vi "ReceiveString.vi"(8 "error in (no error)":errorcluster, 11 "queue cluster":T1) -> (0 "error out":errorcluster, 1 "new value":bool, 2 "received string":string, 3 "queue cluster out":T1)   [LabVIEW 2014]
uses:
  typedefs/clientStatus.ctl
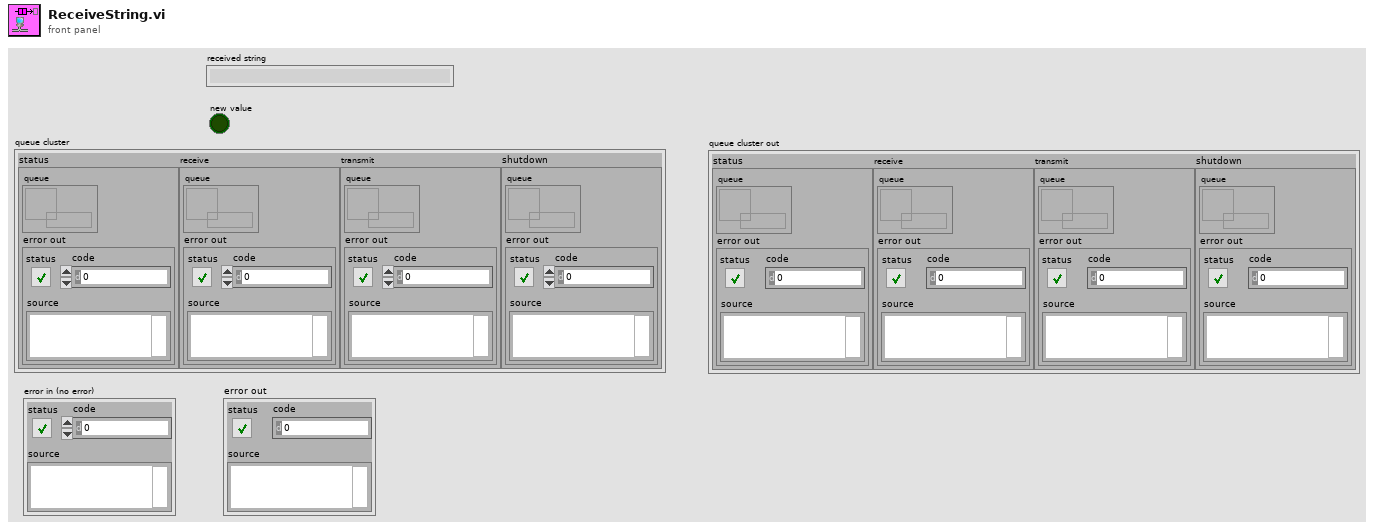
[diagram p1: front panel]
types:
  T1 = cluster{"status":cluster{"queue":refnum<queue>, "error out":errorcluster}, "receive":cluster{"queue":refnum<queue>, "error out":errorcluster}, "transmit":cluster{"queue":refnum<queue>, "error out":errorcluster}, "shutdown":cluster{"queue":refnum<queue>, "error out":errorcluster}}
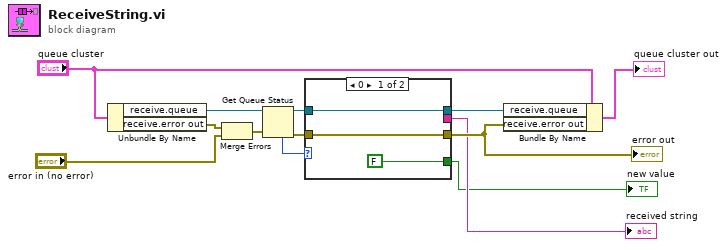
[diagram p0: block diagram]
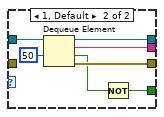
[diagram p2: hidden frame]
diagram:
  n1 = Unbundle By Name("queue cluster") -> ("receive.queue"=w9:refnum<queue>, "receive.error out"=w6:errorcluster)
  n2 = Merge Errors(w6, "error in (no error)") -> (w7:errorcluster)
  n3 = Get Queue Status(queue=w9, error in (no error)=w7) -> (queue out=w8:refnum<queue>, error out=w4:errorcluster, # elements in queue=w3:i32)  [unwired: 1 in, 5 out]
  n4 = case shown="0" w3 {
    tunnel: [w15 w23] -> w11
    tunnel: [w16 w22] -> w10
    tunnel: [_ w21] -> w2
    tunnel: w8 -> [w16 w20]
    tunnel: w4 -> [w15 _]
    tunnel: [FALSE ("timed out?") w17] -> w1
    frame 0 {
    }
    frame 1, Default {
      n5 = Dequeue Element(queue=w20, timeout in ms (-1)=50) -> (queue out=w22:refnum<queue>, element=w21:string, timed out?=w18:bool, error out=w23:errorcluster)  [unwired: 1 in]
      n6 = Not(x=w18) -> (.not. x?=w17:bool)
    }
  }
  "error out" <- w11
  "received string" <- w2
  "new value" <- w1
  n7 = Bundle By Name(cluster="queue cluster", "receive.queue"=w10, "receive.error out"=w11) -> (→"queue cluster out":T1)
